vi "GetRemote with TMO.vi"(4 "error in (no error)":errorcluster, 7 "Timeout, (10000 ms)":u32=10000) -> (0 "error out":errorcluster)   [LabVIEW 2011]
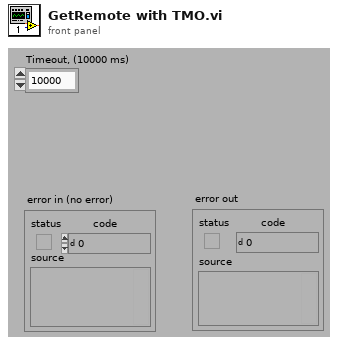
[diagram p1: front panel]
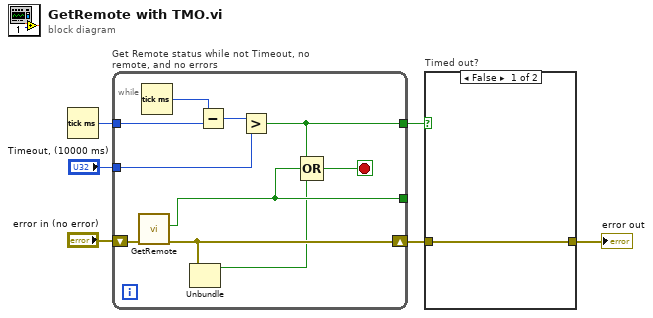
[diagram p0: block diagram]
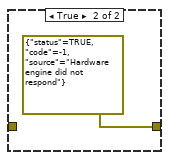
[diagram p2: hidden frame]
diagram:
  n1 = Tick Count (ms)() -> (millisecond timer value=w5:u32)
  n2 = while "Get Remote status while not Timeout, no remote, and no errors" {
    shift-right: [w15] -> w2
    shift-left: "error in (no error)" -> [w16]
    tunnel: [w10] -> _
    tunnel: w5 -> [w14]
    tunnel: "Timeout, (10000 ms)" -> [w11]
    tunnel: [w8] -> w3
    stop <- w7 stop-if-true
    n3 = call "GetRemote.vi"("error in (no error)"=w16) -> ("error out"=w15:errorcluster, "Remote"=w10:bool)  [unwired: 1 in, 8 out]
    n4 = Tick Count (ms)() -> (millisecond timer value=w13:u32)
    n5 = Unbundle(w15) -> ("status"=w9:bool)  [unwired: 2 out]
    n6 = Subtract(x=w13, y=w14) -> (x-y=w12:u32)
    n7 = Greater?(x=w12, y=w11) -> (0:w8:bool)
    n8 = Compound Arithmetic op=OR(w8, w10, w9) -> (w7:bool)
  }
  n9 = case "Timed out?" shown="False" w3 {
    tunnel: w2 -> [w17 _]
    tunnel: [w17 errorcluster {"status"=TRUE, "code"=-1, "source"="Hardware engine did not respond"} ("error in (no error)")] -> w1
    frame False {
    }
    frame True {
    }
  }
  "error out" <- w1
